vi "Experiment header-Update individual internal element values.vi"(9 "Value":dbl, 10 "Name of parameter to update":string, 11 "All params (internal)":T1) -> ()   [LabVIEW 2013]
uses:
  Typedefs/All parameters cluster reference.ctl
  Typedefs/Header parameters cluster-ALL.ctl
  Typedefs/Imaging Protocols enum.ctl
  Typedefs/Frame Size.ctl
  Typedefs/AOL modes.ctl
  Typedefs/Plane Mode.ctl
  Typedefs/Objective selector control enum.ctl
  Typedefs/Header file type enum.ctl
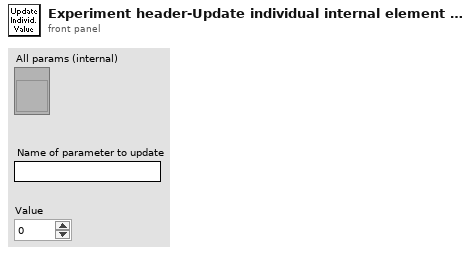
[diagram p1: front panel]
types:
  T1 = typedef "All parameters cluster reference.ctl" = refnum<vi>
  T2 = typedef "Header file type enum.ctl" = enum16{"All parameters", "Params for funct acq w ROI or mscn", "Params for funct acq w rectangles", "Live imaging header parameters", "AOL Parameters"}
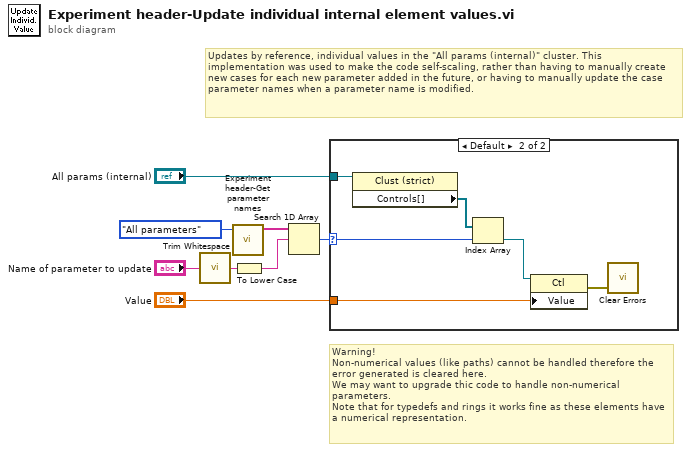
[diagram p0: block diagram]
diagram:
  # "Warning!\nNon-numerical values (like paths) cannot be handled therefore the error generated is cleared here.\nWe may want to upgrade thic code to handle non-numerical parameters.\nNote that for typedefs and rings it works fine as these elements have a numerical representation."
  # "Updates by reference, individual values in the \"All params (internal)\" cluster. This implementation was used to make the code self-scaling, rather than having to manually create new cases for each new parameter added in the future, or having to manually update the case parameter names when a parameter name is modified."
  n1 = call <vilib>:"Trim Whitespace.vi"("string"="Name of parameter to update") -> ("trimmed string"=w5:string)  [unwired: 1 in]
  n2 = call "Experiment header-Get parameter names.vi"("Header file type"=Header_file_type_enum."All parameters") -> ("Parameter names"=w2:string[])  [unwired: 9 in, 1 out]
  n3 = To Lower Case(string=w5) -> (all lower case string=w7:string)
  n4 = Search 1D Array(1D array=w2, element=w7) -> (index of element=w3:i32)  [unwired: 1 in]
  n5 = case shown="Default" w3 {
    selector: w3 -> [_ w14]
    tunnel: "Value" -> [_ w12]
    tunnel: "All params (internal)" -> [_ w9]
    frame -1 {
    }
    frame Default {
      n6 = property on="Property Node" class="Clust (strict)"(reference=w9) -> ("Controls[]"=w10:refnum<vi>[])  [unwired: 1 in, 2 out]
      n7 = Index Array(array=w10, index=w14) -> (element=w13:refnum<vi>)
      n8 = property class="Ctl"(reference=w13, "Value"=w12) -> (error out=w11:errorcluster)  [unwired: 1 in, 1 out]
      n9 = call <vilib>:"Clear Errors.vi"("error in (no error)"=w11) -> ()  [unwired: 6 in, 1 out]
    }
  }
